vi "Make VI Param(Profile Info).vi"(1 "pProfileInfo":T1) -> (0 "Profile Info":T2={"Profile Cnt"=1, "Envelope"=FALSE, " Profile Data Point"=0, " X Start"=0, " X Pitch"=0})   [LabVIEW 2014, in "Keyence LJ-V7000.lvlib"]
uses:
  Keyence LJ-V7000.lvlib
  Public/Clusters/Profile Info.ctl
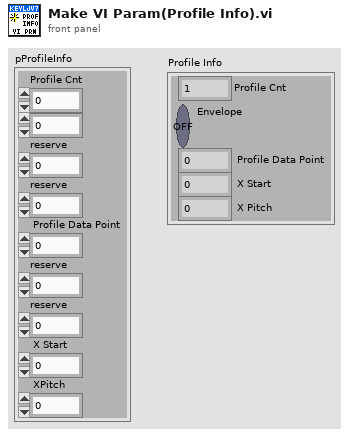
[diagram p1: front panel]
types:
  T1 = cluster{"Profile Cnt":u8, u8, "reserve":u8, "reserve":u8, " Profile Data Point":u16, "reserve":u8, "reserve":u8, " X Start":i32, " XPitch":i32}
  T2 = typedef "Keyence LJ-V7000.lvlib/Profile Info.ctl" = cluster{"Profile Cnt":u8, "Envelope":bool, " Profile Data Point":u16, " X Start":i32, " X Pitch":i32}
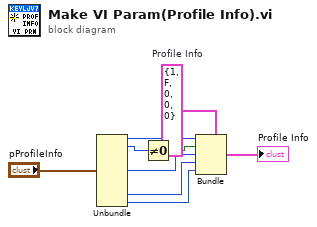
[diagram p0: block diagram]
diagram:
  w6 = T2 {"Profile Cnt"=1, "Envelope"=FALSE, " Profile Data Point"=0, " X Start"=0, " X Pitch"=0}  # Profile Info
  n1 = Unbundle("pProfileInfo") -> ("Profile Cnt"=w2:u8, w3:u8, "Profile Data Point"=w5:u16, "X Start"=w7:i32, "XPitch"=w8:i32)  [unwired: 4 out]
  n2 = Not Equal To 0?(x=w3) -> (x != 0?=w4:bool)
  n3 = Bundle(cluster=w6, "Profile Cnt"=w2, "Envelope"=w4, "Profile Data Point"=w5, "X Start"=w7, "X Pitch"=w8) -> (→"Profile Info":T2)
